vi "init_LS218.vi"(3 "entrée d'erreur":errorcluster caption="sortie d'erreur") -> (0 "sortie d'erreur":errorcluster, 1 "COM_OK":bool, 2 "Nom de ressource VISA en sortie":refnum<visa-resource-name>)   [LabVIEW 2016]
uses:
  <vilib>/Instr/_visa.llb/VISA Set IO Buffer Mask.ctl
  <vilib>/Instr/_visa.llb/VISA Flush IO Buffer Mask.ctl
  <vilib>/Instr/_visa.llb/VISA Configure Serial Port (Instr).vi
panel:
  in  "SET_DATE":bool
  out "Date et heure LSCI218 :":string
  in  "QUITTER":bool
  in  "VALIDER":bool
  in  "CONNECT":bool
  in  "Débit":u32(ring)=9600 items=["1200 Baud"=1200, "9600 Baud"=9600]
  in  "Port COM":refnum<visa-resource-name>="COM8"
  out "Réponse LS218 :":string
  # "ACQUISTION DE TEMPÉRATURE \nLAKE SHORE 218"
  # "J. HANSOTTE - Station d'Étalonnage"
  # "État liaison série :"
  # "Synchronisation date et heure"
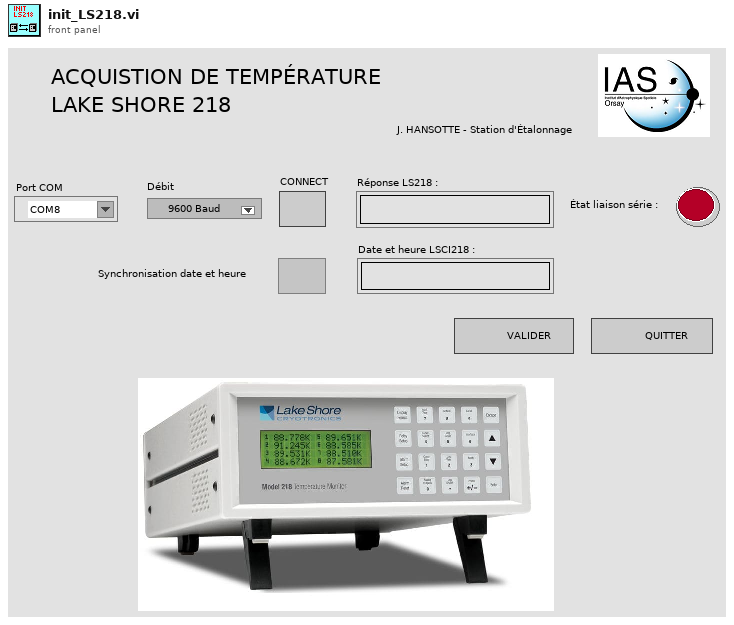
[diagram p1: front panel]
types:
  T1 = enum8{"Enabled", "Disabled", "Disabled and Grayed Out"}
  T2 = typedef "VISA Flush IO Buffer Mask.ctl" = u16
  T3 = typedef "VISA Set IO Buffer Mask.ctl" = u16
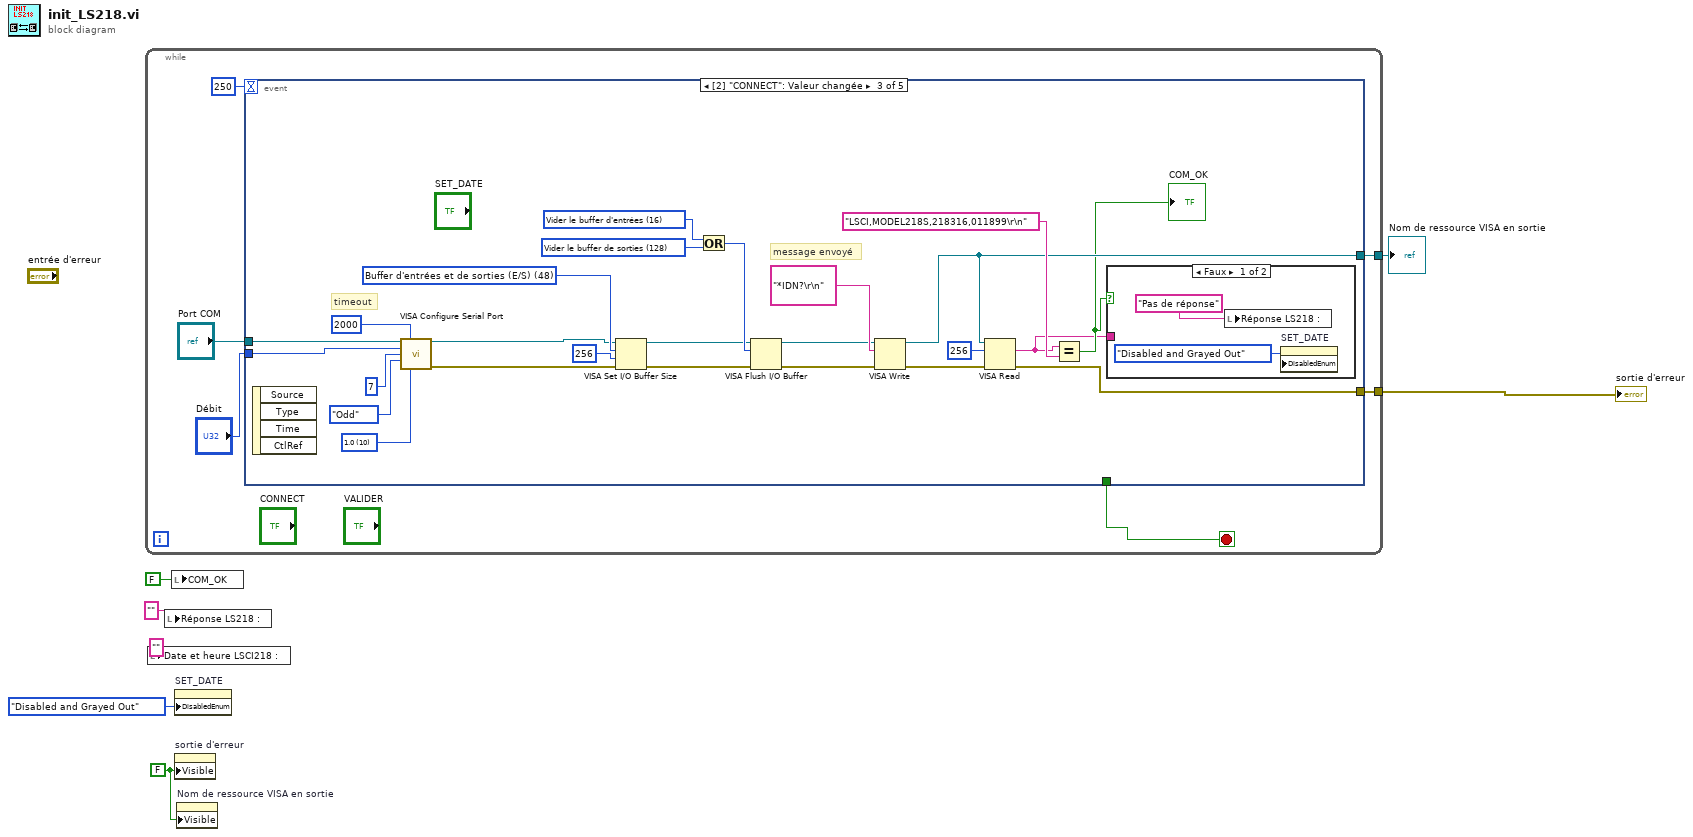
[diagram p0: block diagram]
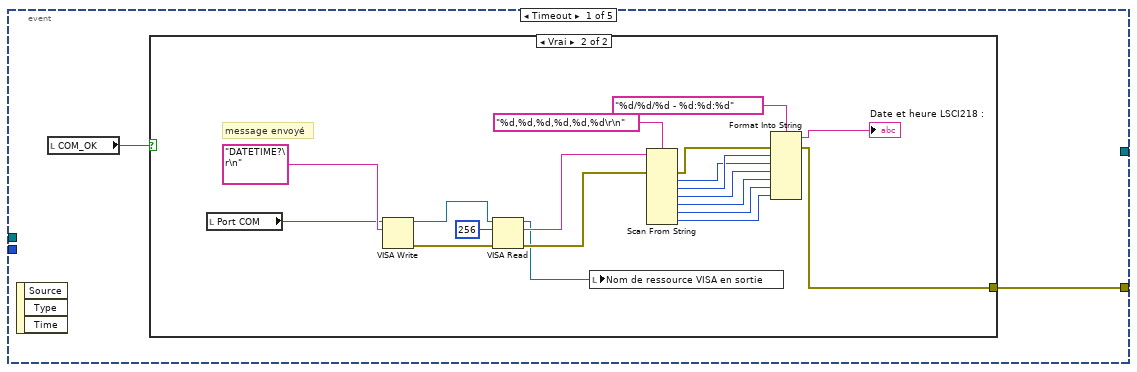
[diagram p2: hidden frame]
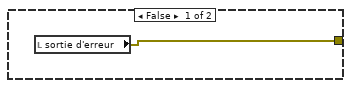
[diagram p3: hidden frame]
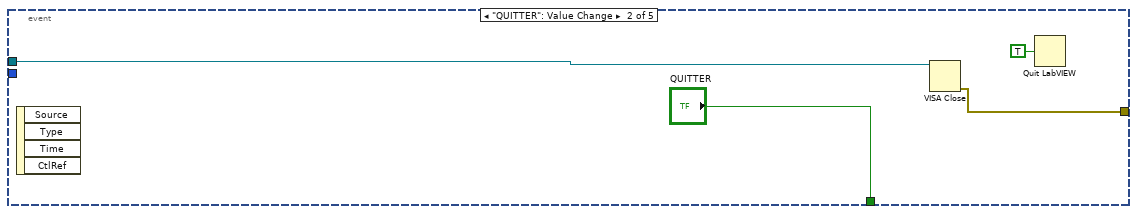
[diagram p4: hidden frame]
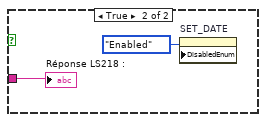
[diagram p5: hidden frame]
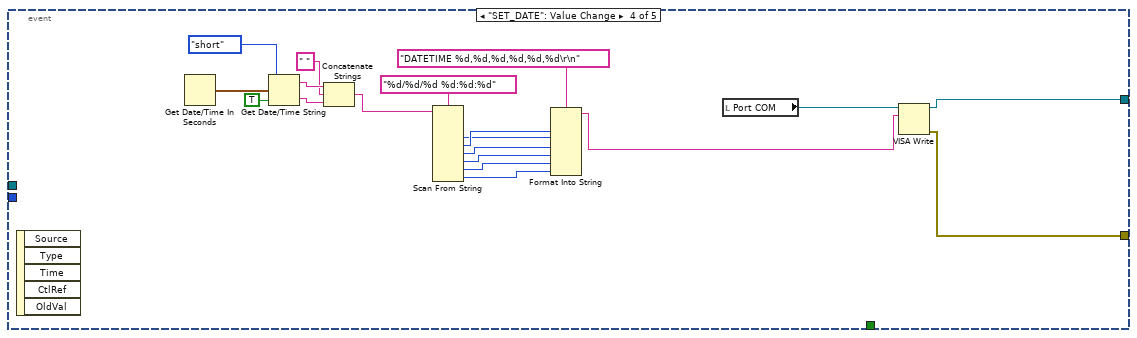
[diagram p6: hidden frame]
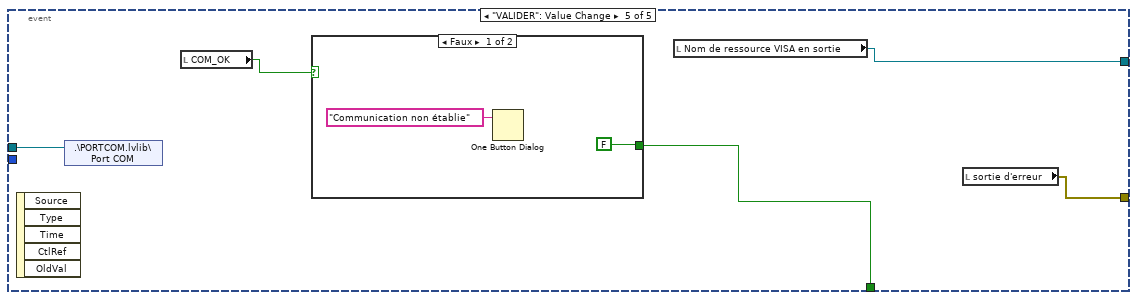
[diagram p7: hidden frame]
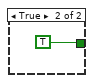
[diagram p8: hidden frame]
diagram:
  w1 = FALSE ("Visible")
  n1 = while {
    tunnel: [w13] -> w6
    tunnel: [w10] -> w5
    stop <- w8 stop-if-true
    n2 = event shown="[2] \"CONNECT\": Valeur changée" {
      selector: _ -> [_ _ _ _ _]
      dyn-events: _ -> [_ _ _ _ _]
      timeout: 250 -> [_ _ _ _ _]
      tunnel: [w14 w37 w43 w86 w92] -> w13
      tunnel: "Port COM" -> [_ w36 w45 _ w88]
      tunnel: "Débit" -> [_ _ w44 _ _]
      tunnel: [_ _ w42 w85 w91] -> w10
      tunnel: [_ "QUITTER" _ _ w90] -> w8
      event Timeout {
        n3 = event-data() -> ()  [unwired: 1 in, 3 out]
        n4 = local read "COM_OK"() -> (w15:bool)
        n5 = case shown="Vrai" w15 {
          tunnel: [w16 w18] -> w14
          frame False {
            n6 = local read "sortie d'erreur"() -> (w16:errorcluster)
          }
          frame True {
            # "message envoyé"
            n7 = local read "Port COM"() -> (w31:refnum<visa-resource-name>)
            n8 = VISA Write(VISA resource name=w31, write buffer="DATETIME?\r\n" ("buffer d'écriture")) -> (VISA resource name out=w32:refnum<visa-resource-name>, error out=w34:errorcluster)  [unwired: 1 in, 1 out]
            n9 = VISA Read(VISA resource name=w32, byte count=u32 256 ("nombre d'octets"), error in (no error)=w34) -> (VISA resource name out=w17:refnum<visa-resource-name>, read buffer=w30:string, error out=w29:errorcluster)  [unwired: 1 out]
            n10 = local write "Nom de ressource VISA en sortie"(w17) -> ()
            n11 = Scan From String(format string="%d,%d,%d,%d,%d,%d\r\n" ("chaîne de format"), input string=w30, error in=w29) -> (error out=w19:errorcluster, output 1=w26:i32, output 2=w27:i32, output 3=w25:i32, output 4=w24:i32, output 5=w23:i32, output 6=w22:i32)  [unwired: 7 in, 2 out]
            n12 = Format Into String(format string="%d/%d/%d - %d:%d:%d" ("chaîne de format"), error in=w19, w27, w26, w25, w24, w23, w22) -> (resulting string=→"Date et heure LSCI218 :":string, error out=w18:errorcluster)  [unwired: 1 in]
          }
        }
      }
      event "QUITTER": Value Change {
        n13 = event-data() -> ()  [unwired: 1 in, 4 out]
        n14 = VISA Close(VISA resource name=w36) -> (error out=w37:errorcluster)  [unwired: 1 in]
        n15 = Quit LabVIEW(quit? (T)=TRUE ("quitter ? (V)")) -> ()
      }
      event "CONNECT": Value Change {
        w64 = u16 10 items=["1.0"=10, "1.5"=15, "2.0"=20] ("stop bits (10: 1 bit)")
        w54 = T2 128 items=["Vider le buffer d'entrées"=16, "Écrire le buffer de sorties sur le périphérique"=32, "Vider le buffer d'entrées (Pas d'E/S)"=64, "Vider le buffer de sorties"=128] ("Mask")
        w53 = T2 16 items=["Vider le buffer d'entrées"=16, "Écrire le buffer de sorties sur le périphérique"=32, "Vider le buffer d'entrées (Pas d'E/S)"=64, "Vider le buffer de sorties"=128] ("Mask")
        w50 = T3 48 items=["Buffer d'entrées (E/S)"=16, "Buffer de sorties (E/S)"=32, "Buffer d'entrées et de sorties (E/S)"=48] ("Mask")
        # "timeout"
        # "message envoyé"
        n16 = event-data() -> ()  [unwired: 1 in, 4 out]
        n17 = call-poly "VISA Configure Serial Port"("VISA resource name"=w45, "timeout (10sec)"=u32 2000, "baud rate (9600)"=w44, "data bits (8)"=u16 7, "parity (0:none)"=enum16{"None", "Odd", "Even", "Mark", "Space"}."Odd", "stop bits (10: 1 bit)"=w64) -> ("VISA resource name out"=w47:refnum<visa-resource-name>, "error out"=w48:errorcluster)  [unwired: 8 in]
        n18 = VISA Set I/O Buffer Size(VISA resource name=w47, mask (16)=w50, size (4096)=u32 256 ("taille (4096)"), error in (no error)=w48) -> (VISA resource name out=w52:refnum<visa-resource-name>, error out=w51:errorcluster)
        n19 = Or(x=w53, y=w54) -> (x .or. y?=w55:T2)
        n20 = VISA Flush I/O Buffer(VISA resource name=w52, mask (16)=w55, error in (no error)=w51) -> (VISA resource name out=w57:refnum<visa-resource-name>, error out=w56:errorcluster)
        n21 = VISA Write(VISA resource name=w57, write buffer="*IDN?\r\n" ("buffer d'écriture"), error in (no error)=w56) -> (VISA resource name out=w42:refnum<visa-resource-name>, error out=w59:errorcluster)  [unwired: 1 out]
        n22 = VISA Read(VISA resource name=w42, byte count=u32 256 ("nombre d'octets"), error in (no error)=w59) -> (read buffer=w40:string, error out=w43:errorcluster)  [unwired: 2 out]
        n23 = Equal?(x=w40, y="LSCI,MODEL218S,218316,011899\r\n") -> (x = y?=w41:bool)
        "COM_OK" <- w41
        n24 = case shown="Faux" w41 {
          tunnel: w40 -> [_ w68]
          frame False {
            n25 = local write "Réponse LS218 :"("Pas de réponse" ("cas faux")) -> ()
            n26 = property on="SET_DATE" class="Bool (strict)"("DisabledEnum"=T1."Disabled and Grayed Out" ("Désactivé")) -> ()  [unwired: 2 in, 2 out]
          }
          frame True {
            n27 = property on="SET_DATE" class="Bool (strict)"("DisabledEnum"=T1."Enabled" ("Désactivé")) -> ()  [unwired: 2 in, 2 out]
            "Réponse LS218 :" <- w68
          }
        }
      }
      event "SET_DATE": Value Change {
        n28 = event-data() -> ()  [unwired: 1 in, 5 out]
        n29 = Get Date/Time In Seconds() -> (seconds since 1Jan1904=w84:timestamp)
        n30 = Get Date/Time String(date format (0)=enum16{"short", "long", "abbreviated"}."short" ("format de date (0)"), seconds (now)=w84, want seconds? (F)=TRUE ("secondes ? (F)")) -> (date string=w81:string, time string=w80:string)
        n31 = Concatenate Strings(w81, " " ("chaîne"), w80) -> (w78:string)
        n32 = Scan From String(format string="%d/%d/%d %d:%d:%d" ("chaîne de format"), input string=w78) -> (output 1=w75:i32, output 2=w76:i32, output 3=w74:i32, output 4=w73:i32, output 5=w72:i32, output 6=w71:i32)  [unwired: 8 in, 3 out]
        n33 = Format Into String(format string="DATETIME %d,%d,%d,%d,%d,%d\r\n" ("chaîne de format"), w76, w75, w74, w73, w72, w71) -> (resulting string=w69:string)  [unwired: 2 in, 1 out]
        n34 = local read "Port COM"() -> (w87:refnum<visa-resource-name>)
        n35 = VISA Write(VISA resource name=w87, write buffer=w69) -> (VISA resource name out=w85:refnum<visa-resource-name>, error out=w86:errorcluster)  [unwired: 1 in, 1 out]
      }
      event "VALIDER": Value Change {
        n36 = event-data() -> ()  [unwired: 1 in, 5 out]
        n37 = shared-variable ".\\PORTCOM.lvlib\\Port COM"(w88) -> ()  [unwired: 1 in, 1 out]
        n38 = local read "COM_OK"() -> (w89:bool)
        n39 = case shown="Faux" w89 {
          tunnel: [FALSE ("Visible") TRUE ("Visible")] -> w90
          frame False {
            n40 = One Button Dialog(message="Communication non établie") -> ()  [unwired: 1 in, 1 out]
          }
          frame True {
          }
        }
        n41 = local read "Nom de ressource VISA en sortie"() -> (w91:refnum<visa-resource-name>)
        n42 = local read "sortie d'erreur"() -> (w92:errorcluster)
      }
    }
  }
  "sortie d'erreur" <- w6
  "Nom de ressource VISA en sortie" <- w5
  n43 = local write "Date et heure LSCI218 :"("" ("Date et heure")) -> ()
  n44 = local write "Réponse LS218 :"("" ("Réponse LS218")) -> ()
  n45 = local write "COM_OK"(FALSE ("COM_OK")) -> ()
  n46 = property on="SET_DATE" class="Bool (strict)"("DisabledEnum"=T1."Disabled and Grayed Out" ("Désactivé")) -> ()  [unwired: 2 in, 2 out]
  n47 = property on="sortie d'erreur" class="Clust (strict)"("Visible"=w1) -> ()  [unwired: 2 in, 2 out]
  n48 = property on="Nom de ressource VISA en sortie" class="NomVISA"("Visible"=w1) -> ()  [unwired: 2 in, 2 out]
